vi "Example - Basic.vi"() -> ()   [LabVIEW 2011]
uses:
  Taskbar Progress Bar.xctl
panel:
  in  "Progress Bar":bool
  out "Taskbar Progress Bar":u64(xcontrol)
  in  "Progress Bar Maximum":u64=100
  # "Taskbar Progress bar  XControl"
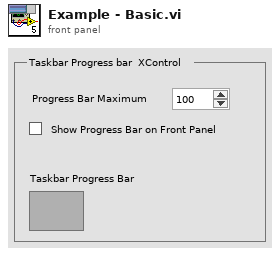
[diagram p1: front panel]
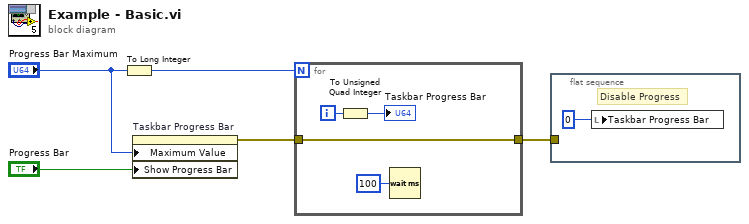
[diagram p0: block diagram]
diagram:
  n1 = To Long Integer(number="Progress Bar Maximum") -> (32bit integer=w4:i32)
  n2 = property on="Taskbar Progress Bar" class="Taskbar Progress Bar (strict)"("Maximum Value"="Progress Bar Maximum", "Show Progress Bar"="Progress Bar") -> (error out=w2:errorcluster)  [unwired: 2 in, 1 out]
  n3 = for {
    N: w4 -> [_]
    tunnel: w2 -> [w6]
    tunnel: [w6] -> w1
    i -> [w8]
    n4 = To Unsigned Quad Integer(1:w8) -> (0:→"Taskbar Progress Bar":u64)
    n5 = Wait (ms)(milliseconds to wait=u32 100) -> ()  [unwired: 1 out]
  }
  n6 = flat-sequence {
    tunnel: w1 -> [_]
    frame #0 {
      # "Disable Progress"
      n7 = local write "Taskbar Progress Bar"(u64 0 ("Taskbar Progress Bar")) -> ()
    }
  }
